vi "Parse APU Array and Resize Prompt.vi"(0 "Tests Array Ref":refnum<vi>, 1 "Controller (Host) Data in":T1, 5 "Selections Array Ref":refnum<vi>, 7 "Done Button Ref":refnum<vi>, 9 "Cancel Button Ref":refnum<vi>, 11 "Prompt VI Ref":refnum<vi>) -> (4 "Scroll Enabled?":bool, 6 "SubTests Array Val":string[](array[string]), 8 "Selection Array Val":bool[](array[boolean]))   [LabVIEW 2018]
uses:
  Public Controls/APU Select.ctl
  Controller (Host).lvlib
  Private Controls/State.ctl
  Private Controls/Controller (Host) Data.ctl
  Top Level/Shared Controls/APU Setup File.ctl
  Public Controls/Test Information.ctl
  Top Level/Shared Controls/Calculated Data.ctl
panel:
  # "Test Information:"
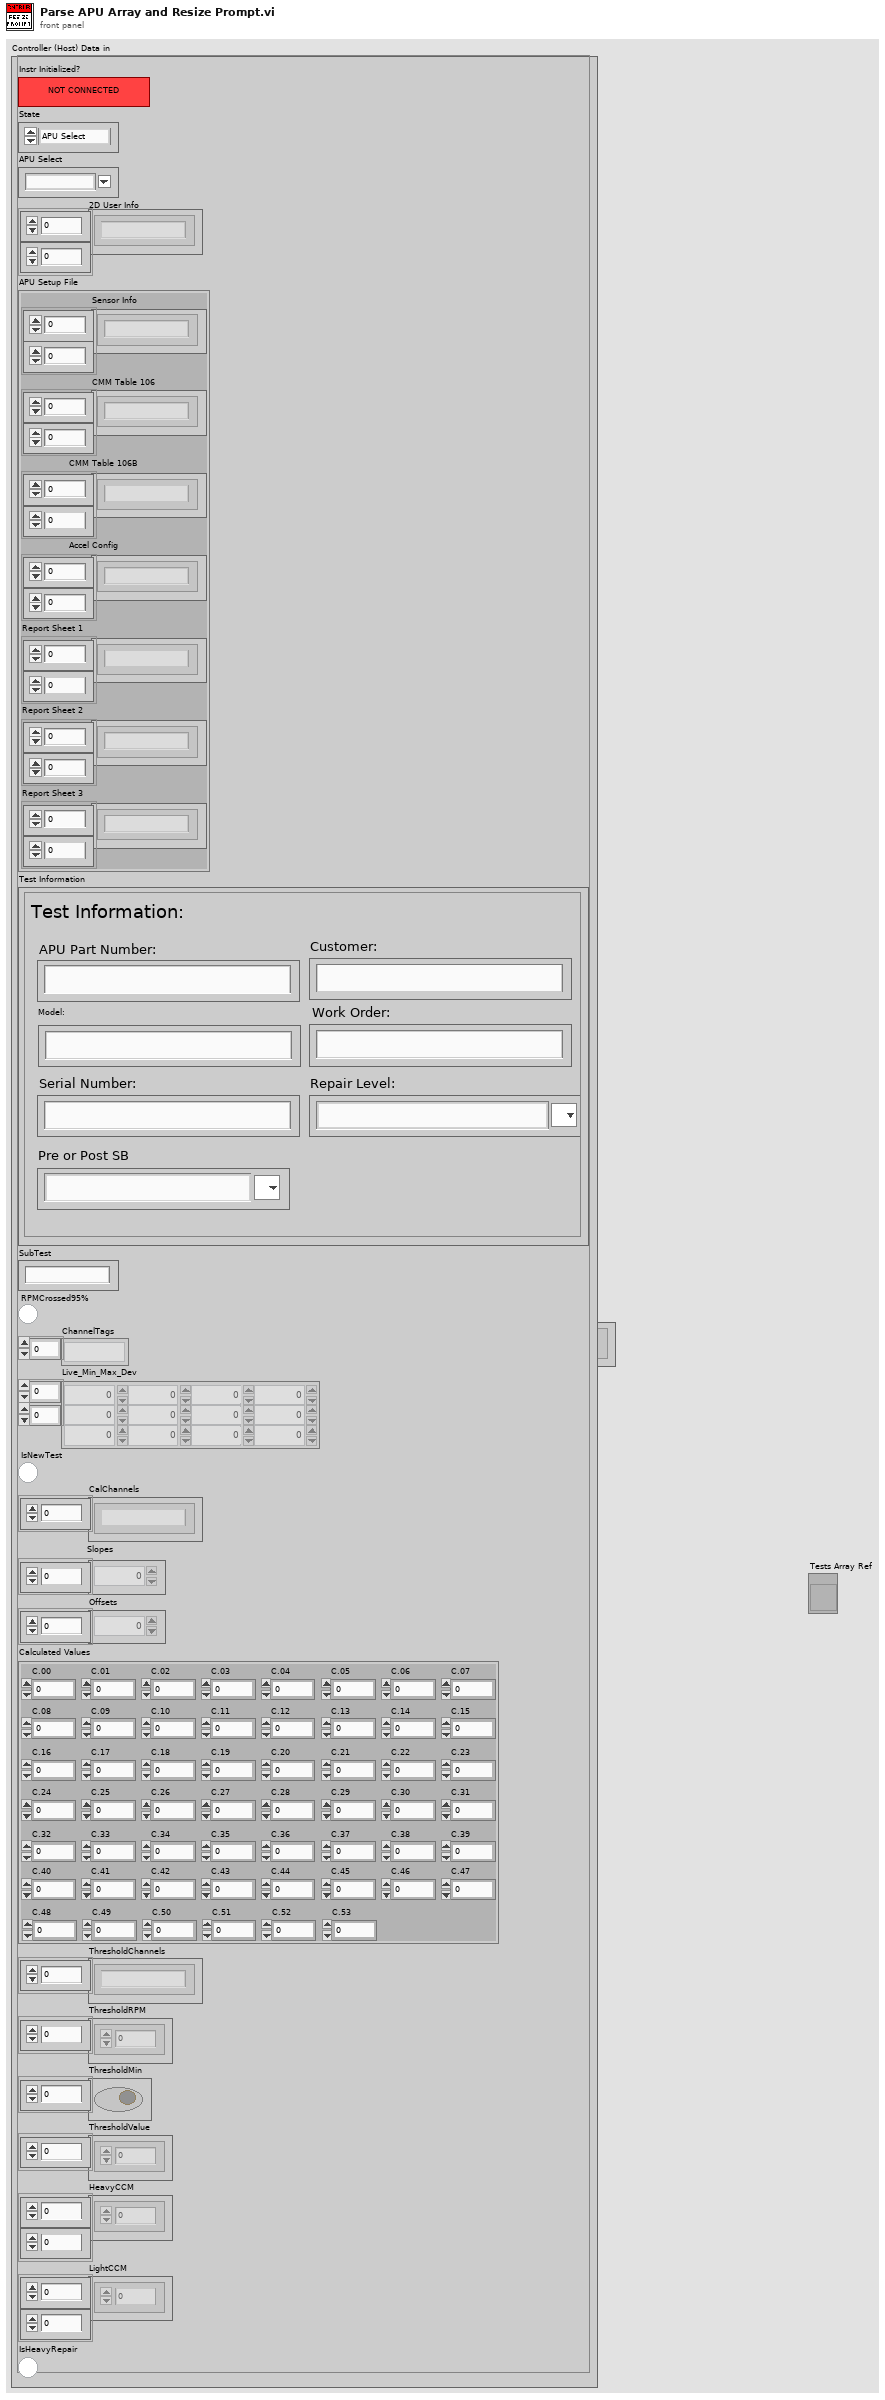
[diagram p1: front panel]
types:
  T1 = typedef "Controller (Host).lvlib/Controller (Host) Data.ctl" = cluster{"Instr Initialized?":bool, "State":T2, "APU Select":T3, "2D User Info":string[][], "APU Setup File":T4, "Test Information":T5, "SubTest":string, "RPMCrossed95%":bool, "ChannelTags":string[], "Live_Min_Max_Dev":dbl[][], "IsNewTest":bool, "CalChannels":string[], "Slopes":dbl[], "Offsets":dbl[], "Calculated Values":T6, "ThresholdChannels":string[], "ThresholdRPM":dbl[], "ThresholdMin":bool[], "ThresholdValue":dbl[], "HeavyCCM":dbl[][], "LightCCM":dbl[][], "IsHeavyRepair":bool}
  T2 = typedef "Controller (Host).lvlib/State.ctl" = enum16{"APU Select", "Operation Select", "SubTests Select", "Calibration", "Testing", "Exit"}
  T3 = typedef "Controller (Host).lvlib/APU Select.ctl" = string
  T4 = typedef "APU Setup File.ctl" = cluster{"Sensor Info":string[][], "CMM Table 106":string[][], "CMM Table 106B ":string[][], "Accel Config":string[][], "Report Sheet 1":string[][], "Report Sheet 2":string[][], "Report Sheet 3":string[][]}
  T5 = typedef "Controller (Host).lvlib/Test Information.ctl" = cluster{"APU Part Number:":string, "Model:":string, "Serial Number:":string, "Customer:":string, "Work Order:":string, "Repair Level:":string, "Pre or Post SB":string}
  T6 = typedef "Calculated Data.ctl" = cluster{"C.00":dbl, "C.01":dbl, "C.02":dbl, "C.03":dbl, "C.04":dbl, "C.05":dbl, "C.06":dbl, "C.07":dbl, "C.08":dbl, "C.09":dbl, "C.10":dbl, "C.11":dbl, "C.12":dbl, "C.13":dbl, "C.14":dbl, "C.15":dbl, "C.16":dbl, "C.17":dbl, "C.18":dbl, "C.19":dbl, "C.20":dbl, "C.21":dbl, "C.22":dbl, "C.23":dbl, "C.24":dbl, "C.25":dbl, "C.26":dbl, "C.27":dbl, "C.28":dbl, "C.29":dbl, "C.30":dbl, "C.31":dbl, "C.32":dbl, "C.33":dbl, "C.34":dbl, "C.35":dbl, "C.36":dbl, "C.37":dbl, "C.38":dbl, "C.39":dbl, "C.40":dbl, "C.41":dbl, "C.42":dbl, "C.43":dbl, "C.44":dbl, "C.45":dbl, "C.46":dbl, "C.47":dbl, "C.48":dbl, "C.49":dbl, "C.50":dbl, "C.51":dbl, "C.52":dbl, "C.53":dbl}
  T7 = typedef "LVRectTypeDef.ctl" = cluster{"Left":i16, "Top":i16, "Right":i16, "Bottom":i16}
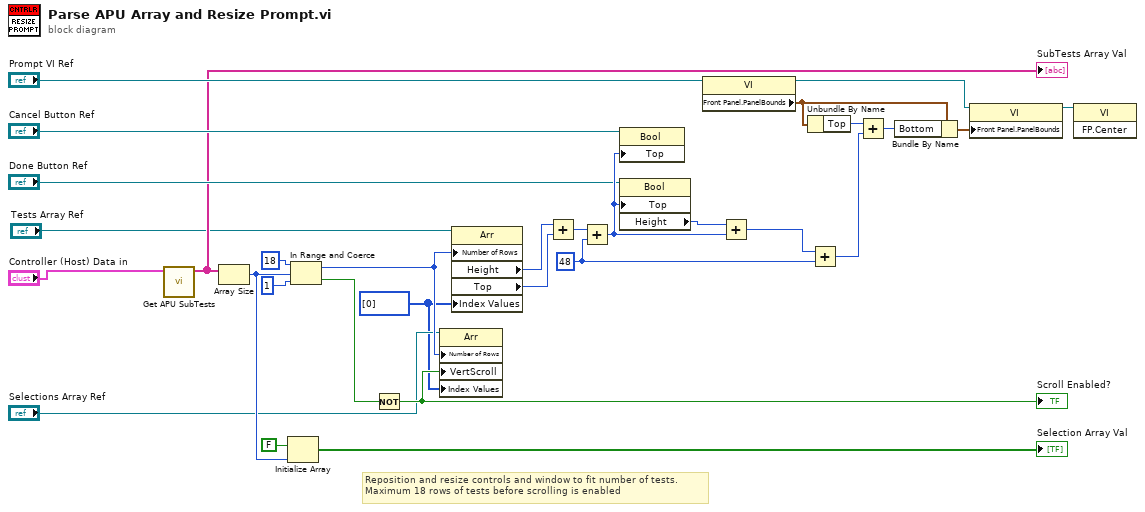
[diagram p0: block diagram]
diagram:
  w3 = u32[] [0] ("Index Values")
  w30 = u32 48 ("y")
  # "Reposition and resize controls and window to fit number of tests.\nMaximum 18 rows of tests before scrolling is enabled"
  n1 = call "Get APU SubTests.vi"("Controller (Host) Data in"="Controller (Host) Data in") -> ("SubTests Array out"=w2:string[])  [unwired: 10 in]
  "SubTests Array Val" <- w2
  n2 = Array Size(array=w2) -> (size(s)=w11:i32)
  n3 = Initialize Array(FALSE, w11) -> (→"Selection Array Val":bool[])
  n4 = In Range and Coerce(upper limit=18, x=w11, lower limit=1) -> (coerced(x)=w12:i32, In Range?=w15:bool)
  n5 = Not(x=w15) -> (.not. x?=w16:bool)
  "Scroll Enabled?" <- w16
  n6 = property on="Property Node" class="Arr"(reference="Selections Array Ref", "Number of Rows"=w12, "VertScroll"=w16, "Index Values"=w3) -> ()  [unwired: 1 in, 2 out]
  n7 = property on="Property Node" class="Arr"(reference="Tests Array Ref", "Number of Rows"=w12, "Index Values"=w3) -> ("Height"=w17:u32, "Top"=w18:i32)  [unwired: 1 in, 2 out]
  n8 = Add(x=w17, y=w18) -> (x+y=w19:u32)
  n9 = Add(x=w19, y=w30) -> (x+y=w21:u32)
  n10 = property on="Property Node" class="Bool"(reference="Cancel Button Ref", "Top"=w21) -> ()  [unwired: 1 in, 2 out]
  n11 = property on="Property Node" class="Bool"(reference="Done Button Ref", "Top"=w21) -> ("Height"=w20:u32)  [unwired: 1 in, 2 out]
  n12 = property class="VI"(reference="Prompt VI Ref") -> (reference out=w23:refnum<vi>, "Front Panel.PanelBounds"=w25:T7)  [unwired: 1 in, 1 out]
  n13 = Add(x=w20, y=w21) -> (x+y=w28:u32)
  n14 = Unbundle By Name(w25) -> ("Top"=w26:i16)
  n15 = Add(x=w28, y=w30) -> (x+y=w29:u32)
  n16 = Add(x=w26, y=w29) -> (x+y=w27:u32)
  n17 = Bundle By Name(cluster=w25, "Bottom"=w27) -> (w24:T7)
  n18 = property class="VI"(reference=w23, "Front Panel.PanelBounds"=w24) -> (reference out=w4:refnum<vi>)  [unwired: 1 in, 1 out]
  n19 = invoke class="VI" method="FP.Center"(reference=w4) -> ()  [unwired: 2 in, 3 out]
